vi "DisabledColorGlobal.vi"() -> ()   [LabVIEW 2013]
panel:
  in  "Disable Color":u32(colorbox)=13816530
  # "To change color, click box and choose.\nThen Edit->Make Current Values Default...\nand Save."
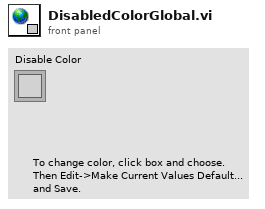
[diagram p1: front panel]
diagram:
